vi "SteeringValidate.vi"() -> ()   [LabVIEW 2016]
uses:
  <vilib>/Platform/TimedLoop/XDataNode/timing_clust.ctl
  <vilib>/Platform/TimedLoop/XDataNode/nitl_modes.ctl
  <vilib>/Platform/TimedLoop/XDataNode/wakeup.ctl
  <vilib>/FPGAPlugInAG/roboRIO/niLvFpga_Open_roboRIO.vi
  <vilib>/rvi/interface/common/dynamic/niFpgaDynamicAddResources.vi
  <vilib>/FPGAPlugInAG/Dynamic/niLvFpga_Reset_Dynamic.vi
  <vilib>/FPGAPlugInAG/Dynamic/niLvFpga_Run_Dynamic.vi
  <vilib>/Utility/error.llb/Error Cluster From Error Code.vi
  <vilib>/rvi/errors/niLvFpgaAdjustHostInterfaceError.vi
  <vilib>/FPGAPlugInAG/Dynamic/niLvFpga_Abort_Dynamic.vi
  <vilib>/FPGAPlugInAG/Dynamic/niLvFpga_Close_Dynamic.vi
  <vilib>/rvi/interface/nirviOpenFPGA/nirviOpenFPGA.xnode
  FPGA Bitfiles/AutoBikeProject_FPGATarget_FPGASteeringVali_0ktHJXMggMw.lvbitx
  <vilib>/rvi/interface/nirviMethod/nirviMethod.xnode
  <vilib>/Platform/TimedLoop/XDataNode/XDataNode.xnode
  <vilib>/rvi/interface/nirviReadWriteControl/nirviReadWriteControl.xnode
  <vilib>/rvi/interface/nirviCloseFPGA/nirviCloseFPGA.xnode
  <vilib>/Platform/TimedLoop/XDataNode/XDNodeRunTimeDep.lvlib
  <vilib>/rvi/interface/Simulation/niFpgaSimulationCallBeginRW.vi
  NiFpgaLv.dll
panel:
  in  "Reset steering angle":bool
  out "Finished Late? [i-1]":bool
  in  "Stop":bool
  out "RPM":dbl
  in  "Frequency of duty cycle":u32=40000
  in  "Direction":bool
  out "Steering angle(deg)":dbl
  in  "RPM":dbl step=1.0
  out "error out":errorcluster
  in  "error in (no error)":errorcluster
  # "Front Panel Controls"
  # "CC"
  # "CW"
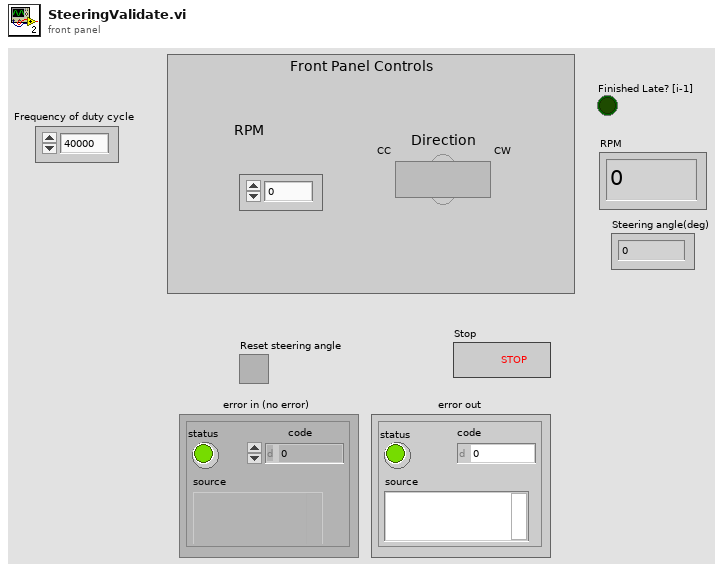
[diagram p1: front panel]
types:
  T1 = enum16{"open", "open or create", "create or replace", "create", "open (read-only)"}
  T2 = typedef "XDNodeRunTimeDep.lvlib/timing_clust.ctl" = cluster{"Expected End [f-1]":u64, "Actual End [f-1]":u64, "Finished Late? [f-1]":bool, "Expected End [i-1]":u64, "Actual End [i-1]":u64, "Finished Late? [i-1]":bool, "Expected Start [i]":u64, "Actual Start [i]":u64, "Expected Start [f]":u64, "Actual Start [f]":u64, "Source Name":string, "Structure Name":string, "Period":i64, "Deadline":i64, "Offset":i64, "Start":i64, "Priority":i32, "Timeout":i32, "Mode":T3, "Wakeup Reason":T4, "Error":errorcluster, "Source Type":string, "Secondary Source Type":string, "Global End Time":u64, "Global Start Time":u64, "Frame Duration":u64, "Iteration Duration":u64, "Assigned CPU":i32, "I/O Scan Engine Mode":u32}
  T3 = typedef "XDNodeRunTimeDep.lvlib/nitl_modes.ctl" = enum32{"No Change", "Process missed periods, maintain original phase", "Discard missed periods, maintain original phase", "Process missed periods, ignore original phase", "Discard missed periods, ignore original phase"}
  T4 = typedef "XDNodeRunTimeDep.lvlib/wakeup.ctl" = enum32{"Normal", "Aborted", "Asynchronous wakeup", "Timing source error", "Timed loop error", "Timeout"}
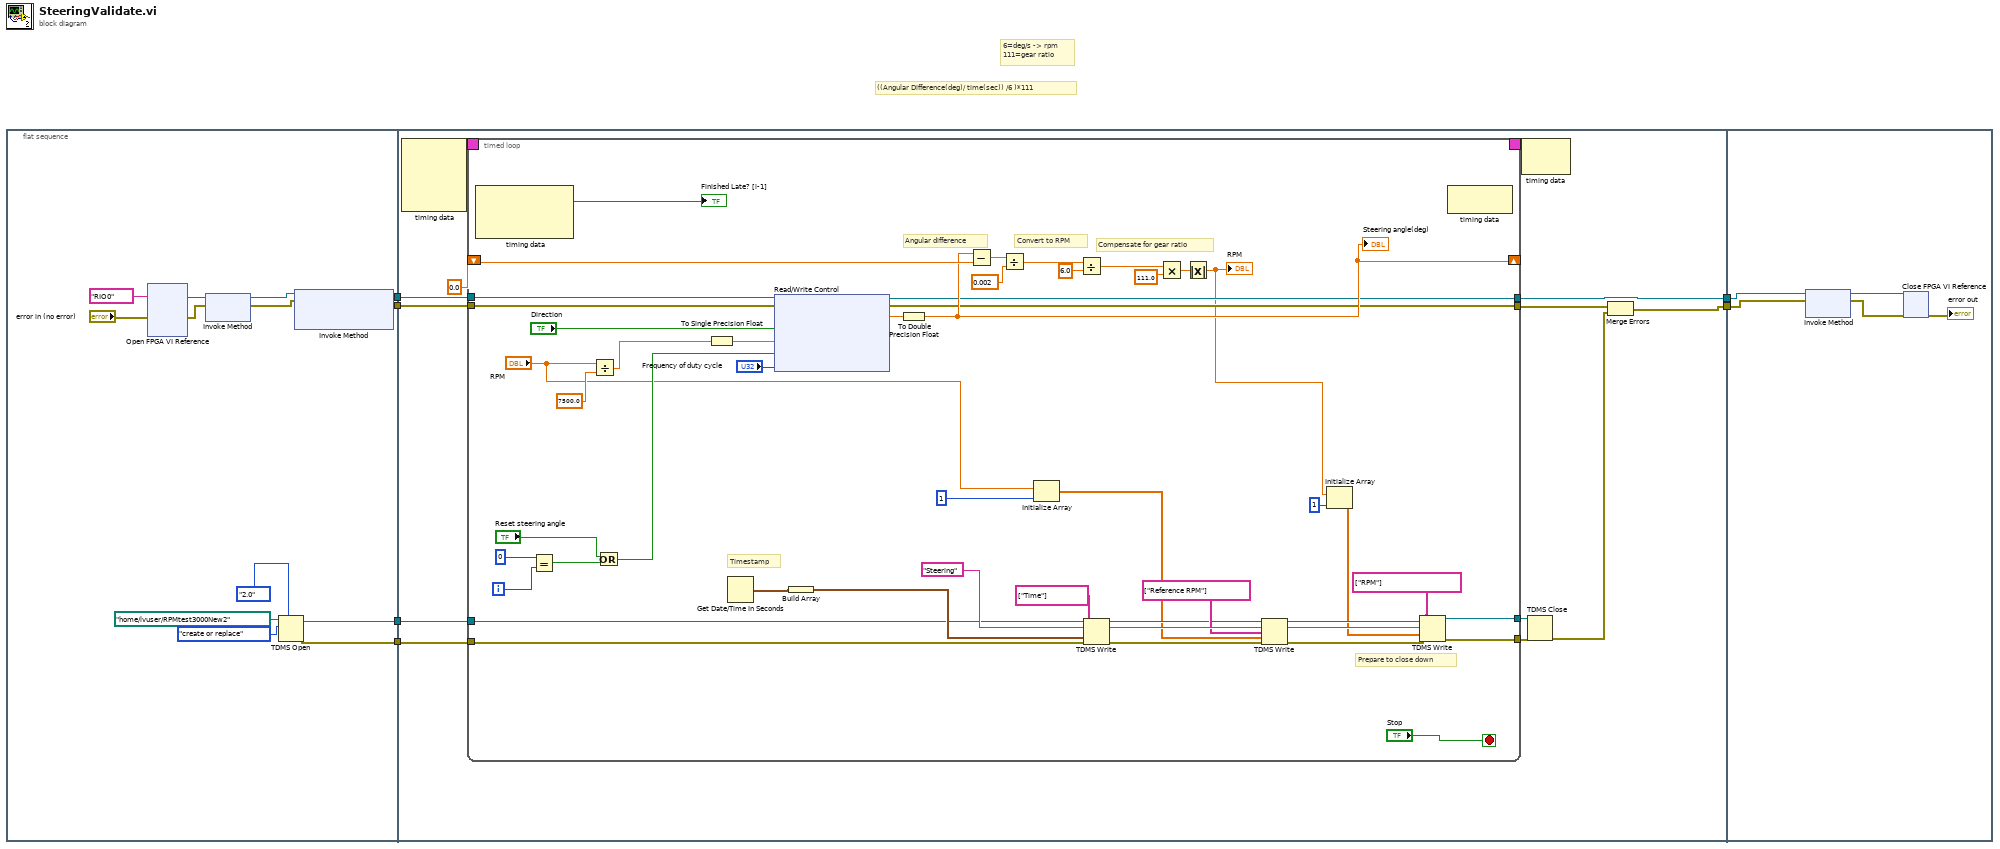
[diagram p0: block diagram]
diagram:
  # "6=deg/s -> rpm\n111=gear ratio"
  # "((Angular Difference(deg)/ time(sec)) /6 )*111"
  n1 = flat-sequence {
    tunnel: [w10] -> w6
    tunnel: [w9] -> w5
    tunnel: [w12] -> w4
    tunnel: [w11] -> w3
    tunnel: w6 -> [w29]
    tunnel: w5 -> [w28]
    tunnel: w4 -> [w27]
    tunnel: w3 -> [w26]
    tunnel: [w30] -> w2
    tunnel: [w25] -> w1
    tunnel: w2 -> [w87]
    tunnel: w1 -> [w86]
    frame #0 {
      n2 = xnode "Open FPGA VI Reference"("error in"="error in (no error)", "resource name"=tag "RIO0") -> ("FPGA VI Reference Out"=w17:refnum<k20>, "error out"=w16:errorcluster)
      n3 = xnode "Invoke Method"("FPGA VI Reference In"=w17, "error in"=w16) -> ("FPGA VI Reference Out"=w7:refnum<k20>, "error out"=w8:errorcluster)
      n4 = TDMS Open(7:enum16{"1.0", "2.0"}."2.0" ("file format version (2.0)"), 10:T1."create or replace" ("operation (0:open)"), 11:path "/home/lvuser/RPMtest3000New2" ("file path")) -> (0:w11:errorcluster, 3:w12:refnum<k34>)  [unwired: 4 in]
      n5 = xnode "Invoke Method"("FPGA VI Reference In"=w7, "error in"=w8) -> ("FPGA VI Reference Out"=w10:refnum<k20>, "error out"=w9:errorcluster)  [unwired: 1 in]
    }
    frame #1 {
      n6 = node-c288() -> (w32:T2)  [unwired: 4 in]
      n7 = timed-loop {
        timing: w32 -> [_]
        timing-out: [_] -> w31
        tunnel: [w42] -> w30
        tunnel: [w41] -> w24
        tunnel: w29 -> [w80]
        tunnel: w28 -> [w79]
        tunnel: w27 -> [w68]
        tunnel: w26 -> [w67]
        tunnel: [w64] -> w23
        tunnel: [w63] -> w22
        shift-right: [w45] -> _
        shift-left: 0.0 -> [w57]
        i -> [w58]
        stop <- "Stop" stop-if-true
        # "Prepare to close down"
        # "Timestamp"
        # "Compensate for gear ratio"
        # "Convert to RPM"
        # "Angular difference"
        n8 = node-c288() -> (→"Finished Late? [i-1]":bool)  [unwired: 1 in, 2 out]
        n9 = Equal?(x=0, y=w58) -> (x = y?=w38:bool)
        n10 = Divide(x="RPM", y=7500.0) -> (x/y=w48:dbl)
        n11 = Or(x="Reset steering angle", y=w38) -> (x .or. y?=w37:bool)
        n12 = To Single Precision Float(number=w48) -> (single precision float=w49:sgl)
        n13 = Get Date/Time In Seconds() -> (seconds since 1Jan1904=w78:timestamp)
        n14 = xnode "Read/Write Control"("FPGA VI Reference In"=w80, "error in"=w79, "Direction"="Direction", "Front Panel Duty Cycle"=w49, "Reset counter"=w37, "Freq"="Frequency of duty cycle") -> ("FPGA VI Reference Out"=w42:refnum<k20>, "error out"=w41:errorcluster, "Steering angle(deg)"=w50:sgl)
        n15 = Build Array(w78) -> (w77:timestamp[])
        n16 = To Double Precision Float(number=w50) -> (double precision float=w45:dbl)
        "Steering angle(deg)" <- w45
        n17 = Subtract(x=w45, y=w57) -> (x-y=w56:dbl)
        n18 = Divide(x=w56, y=0.002) -> (x/y=w53:dbl)
        n19 = Initialize Array("RPM", 1 ("dimension size")) -> (w52:dbl[])
        n20 = Divide(x=w53, y=6.0) -> (x/y=w47:dbl)
        n21 = TDMS Write(0:w68, 5:"Steering" ("group name in (Untitled)"), 7:string[] ["Time"] ("channel name(s) in (Untitled)"), 9:w77, 11:w67) -> (4:w69:refnum<k34>, 6:w74:string, 15:w66:errorcluster)  [unwired: 1 in, 1 out]
        n22 = Multiply(x=w47, y=111.0) -> (x*y=w44:dbl)
        n23 = Absolute Value(x=w44) -> (abs(x)=w39:dbl)
        "RPM" <- w39
        n24 = TDMS Write(0:w69, 5:w74, 7:string[] ["Reference RPM"] ("channel name(s) in (Untitled)"), 9:w52, 11:w66) -> (4:w70:refnum<k34>, 6:w72:string, 15:w65:errorcluster)  [unwired: 1 in, 1 out]
        n25 = Initialize Array(w39, 1 ("dimension size")) -> (w55:dbl[])
        n26 = TDMS Write(0:w70, 5:w72, 7:string[] ["RPM"] ("channel name(s) in (Untitled)"), 9:w55, 11:w65) -> (4:w63:refnum<k34>, 15:w64:errorcluster)  [unwired: 1 in, 2 out]
        n27 = node-c288() -> ()  [unwired: 1 in, 1 out]
      }
      n28 = node-c288(w31) -> ()  [unwired: 1 out]
      n29 = TDMS Close(8:w23, 11:w22) -> (0:w21:errorcluster)  [unwired: 1 out]
      n30 = Merge Errors(w24, w21) -> (w25:errorcluster)
    }
    frame #2 {
      n31 = xnode "Invoke Method"("FPGA VI Reference In"=w87, "error in"=w86) -> ("FPGA VI Reference Out"=w89:refnum<k20>, "error out"=w90:errorcluster)
      n32 = xnode "Close FPGA VI Reference"("FPGA VI Reference In"=w89, "error in"=w90) -> ("error out"=→"error out":errorcluster)
    }
  }
